vi "LogData.vi"(8 "거리 배열":dbl[](array[numeric]), 9 "스톡스 배열":dbl[](array[numeric]), 10 "안티스톡스 배열":dbl[](array[numeric]), 11 "데이터 총량":u32) -> (0 "LOG(AS)-LOG(S)":dbl[](array[numeric]), 1 "LOG(AS-S)":dbl[](array[numeric]), 2 "LOG(S)":dbl[](array[numeric]), 3 "LOG(AS)":dbl[](array[numeric]))   [LabVIEW 2020]
panel:
  out "XY Graph":cluster{"Y":dbl[], "Y":dbl[]}[](graph) caption="XY 그래프"
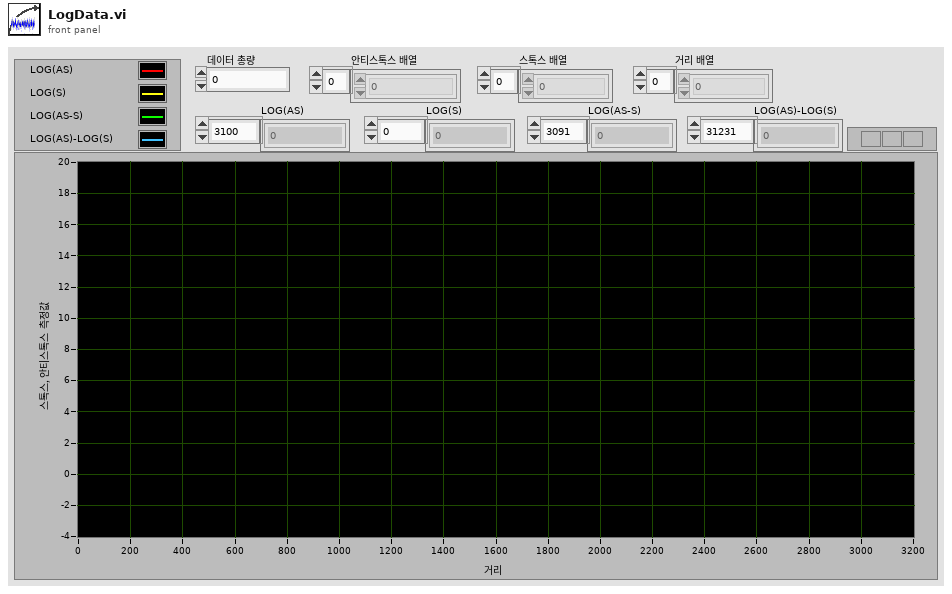
[diagram p1: front panel]
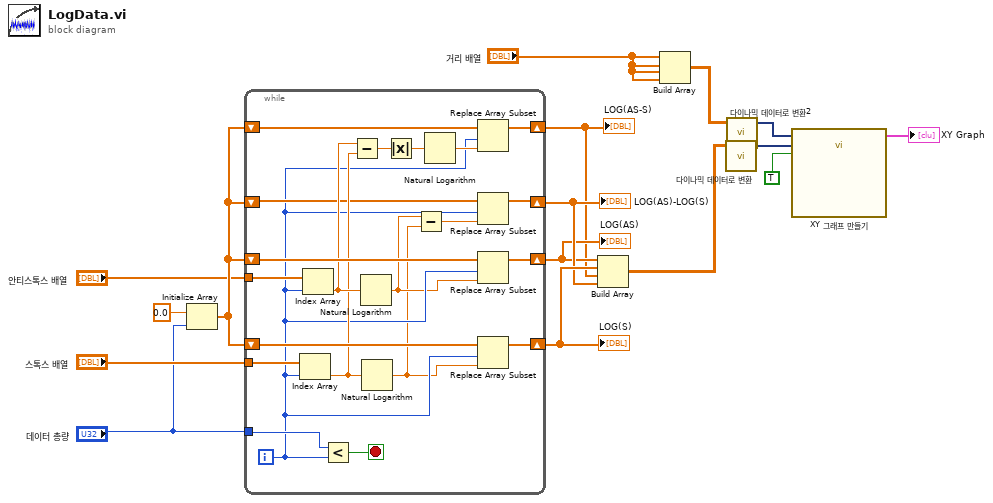
[diagram p0: block diagram]
diagram:
  n1 = Initialize Array(0.0 ("원소"), "데이터 총량") -> (w9:dbl[])
  n2 = while {
    tunnel: "데이터 총량" -> [w37]
    shift-right: [w34] -> w2
    shift-left: w9 -> [w35]
    shift-right: [w33] -> w12
    shift-left: w9 -> [w32]
    tunnel: "안티스톡스 배열" -> [w31]
    tunnel: "스톡스 배열" -> [w30]
    shift-right: [w27] -> w1
    shift-left: w9 -> [w26]
    shift-right: [w24] -> w4
    shift-left: w9 -> [w23]
    i -> [w22]
    stop <- w36 stop-if-true
    n3 = Index Array(array=w30, index=w22) -> (element=w28:dbl)
    n4 = Index Array(array=w31, index=w22) -> (element=w29:dbl)
    n5 = Less?(x=w37, y=w22) -> (x < y?=w36:bool)
    n6 = Subtract(x=w29, y=w28) -> (x-y=w19:dbl)
    n7 = Natural Logarithm(1:w29) -> (0:w21:dbl)
    n8 = Natural Logarithm(1:w28) -> (0:w20:dbl)
    n9 = Absolute Value(x=w19) -> (abs(x)=w18:dbl)
    n10 = Subtract(x=w21, y=w20) -> (x-y=w17:dbl)
    n11 = Natural Logarithm(1:w18) -> (0:w25:dbl)
    n12 = Replace Array Subset(array=w26, new element=w25, index=w22) -> (w27:dbl[])
    n13 = Replace Array Subset(array=w23, new element=w17, index=w22) -> (w24:dbl[])
    n14 = Replace Array Subset(array=w35, new element=w21, index=w22) -> (w34:dbl[])
    n15 = Replace Array Subset(array=w32, new element=w20, index=w22) -> (w33:dbl[])
  }
  "LOG(AS-S)" <- w1
  "LOG(AS)-LOG(S)" <- w4
  "LOG(S)" <- w12
  "LOG(AS)" <- w2
  n16 = Build Array(w2, w12, w1, w4) -> (w11:dbl[][])
  n17 = Build Array("거리 배열", "거리 배열", "거리 배열", "거리 배열") -> (w8:dbl[][])
  n18 = call "다이나믹 데이터로 변환"("2D Array"=w11) -> ("Dynamic Data Type"=w14:dynamicdata)  [unwired: 3 in]
  n19 = call "다이나믹 데이터로 변환2"("2D Array"=w8) -> ("Dynamic Data Type"=w15:dynamicdata)  [unwired: 3 in]
  n20 = call "XY 그래프 만들기"("Reset"=TRUE, "Y Input"=w14, "X Input"=w15) -> ("XY Graph"=→"XY Graph":cluster{"X":dbl[], "Y":dbl[]}[])  [unwired: 7 in, 1 out]
